vi "Unnitialize Shift Register.vi"() -> ()   [LabVIEW 2015]
panel:
  out "Data":u32
  out "Iterasi":u32
  out "Out":u32
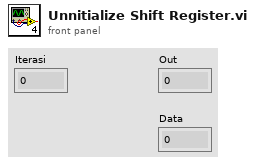
[diagram p1: front panel]
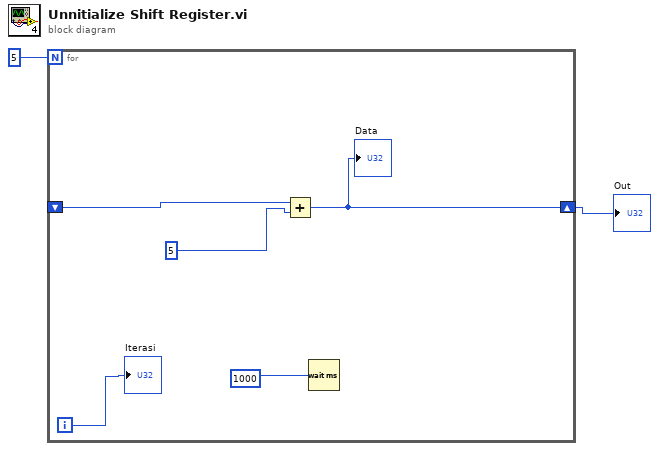
[diagram p0: block diagram]
diagram:
  n1 = for {
    N: 5 -> [_]
    shift-right: [w3] -> w2
    shift-left: _ -> [w4]
    i -> [w5]
    n2 = Add(x=w4, y=5) -> (x+y=w3:i32)
    "Data" <- w3
    n3 = Wait (ms)(milliseconds to wait=1000) -> ()  [unwired: 1 out]
    "Iterasi" <- w5
  }
  "Out" <- w2
